vi "Main.vi"(0 "Operations Combo Box":string(combo)="Add", 1 "Load":bool, 5 "Add":bool, 7 "Delete":bool, 9 "Save":bool, 11 "error in":errorcluster, 12 "Tree":string(tree)) -> (15 "error out":errorcluster)   [LabVIEW 2023]
doc: "This is a simple calculator which can perform basic arithmetic operations like add, subtract, multiply and divide."
uses:
  Typedef/ClassClusters.ctl
  Arithmetic/Arithmetic.lvclass
  Typedef/InstancesArray.ctl
  Typedef/DVRcluster.ctl
  Typedef/DVRInstances.ctl
  Typedef/OperationsCluster.ctl
  Typedef/QueueOperations.ctl
  <vilib>/Utility/xml.llb/Write to XML File(string).vi
  <vilib>/Utility/xml.llb/Read From XML File(array).vi
panel:
  # "CALCULATOR"
  # "INSTRUCTIONS\n\n1. Run the VI.\n2. Choose the operations to perform from the Operations Combo Box.\n3. Press ADD to display once instance of the operations in the Tree.\n4. Press any instances in the tree to load that particular operations in \n    the subpanel.\n5. In the Sub-panel enter the inputs and press CALCULATE to get the \n     output.\n6. Press SAVE to save the operations data in the XML file.\n7. Press LOAD to retrive the save data from the XML, and press the saved\n    instance in the tree to display in the subpanel.\n8. Select any instance and press DELETE to reove from the tree.\n9. Close the Front panel to abort the VI."
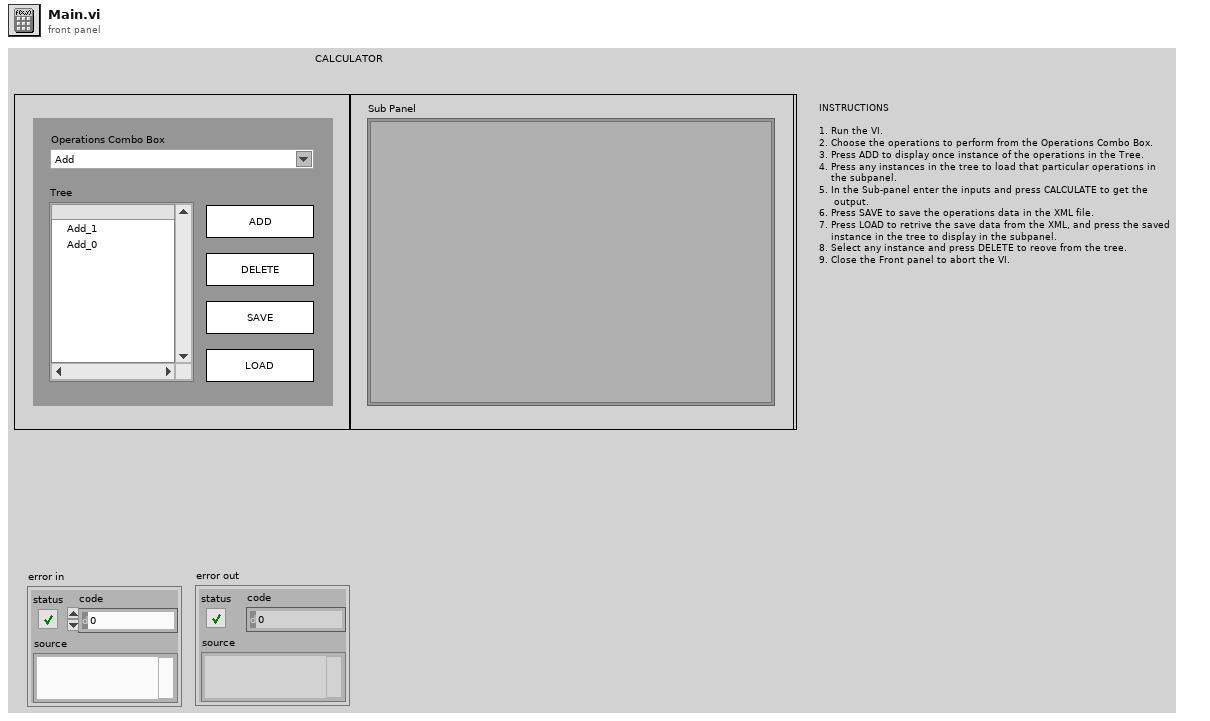
[diagram p1: front panel]
types:
  T1 = typedef "QueueOperations.ctl" = enum16{"Create", "Enqueue", "Enqueue N elements", "Dequeue", "Flush", "Release"}
  T2 = typedef "ClassClusters.ctl" = cluster{"Check":bool, "Combo Box":string, "Add":bool, "Delete":bool, "Path":path, "Tag":string, "Operation data":refnum<class "Arithmetic.lvclass">, "Instances Array":T3[], "XML path":path, "DVR":T4, "Operations Data":T6}
  T3 = typedef "InstancesArray.ctl" = cluster{"Tag":string, "Operation data":refnum<class "Arithmetic.lvclass">}
  T4 = typedef "DVRcluster.ctl" = cluster{"data value reference out":refnum<data-value>, "Operation Data DVR":refnum<data-value>, "Instances Array DVR":T5[]}
  T5 = typedef "DVRInstances.ctl" = cluster{"Operation Data DVR":refnum<data-value>, "Tag":string}
  T6 = typedef "OperationsCluster.ctl" = cluster{"A":dbl, "B":dbl, "C":dbl}
  T7 = typedef "LVPoint32TypeDef.ctl" = cluster{"Horizontal":i32, "Vertical":i32}
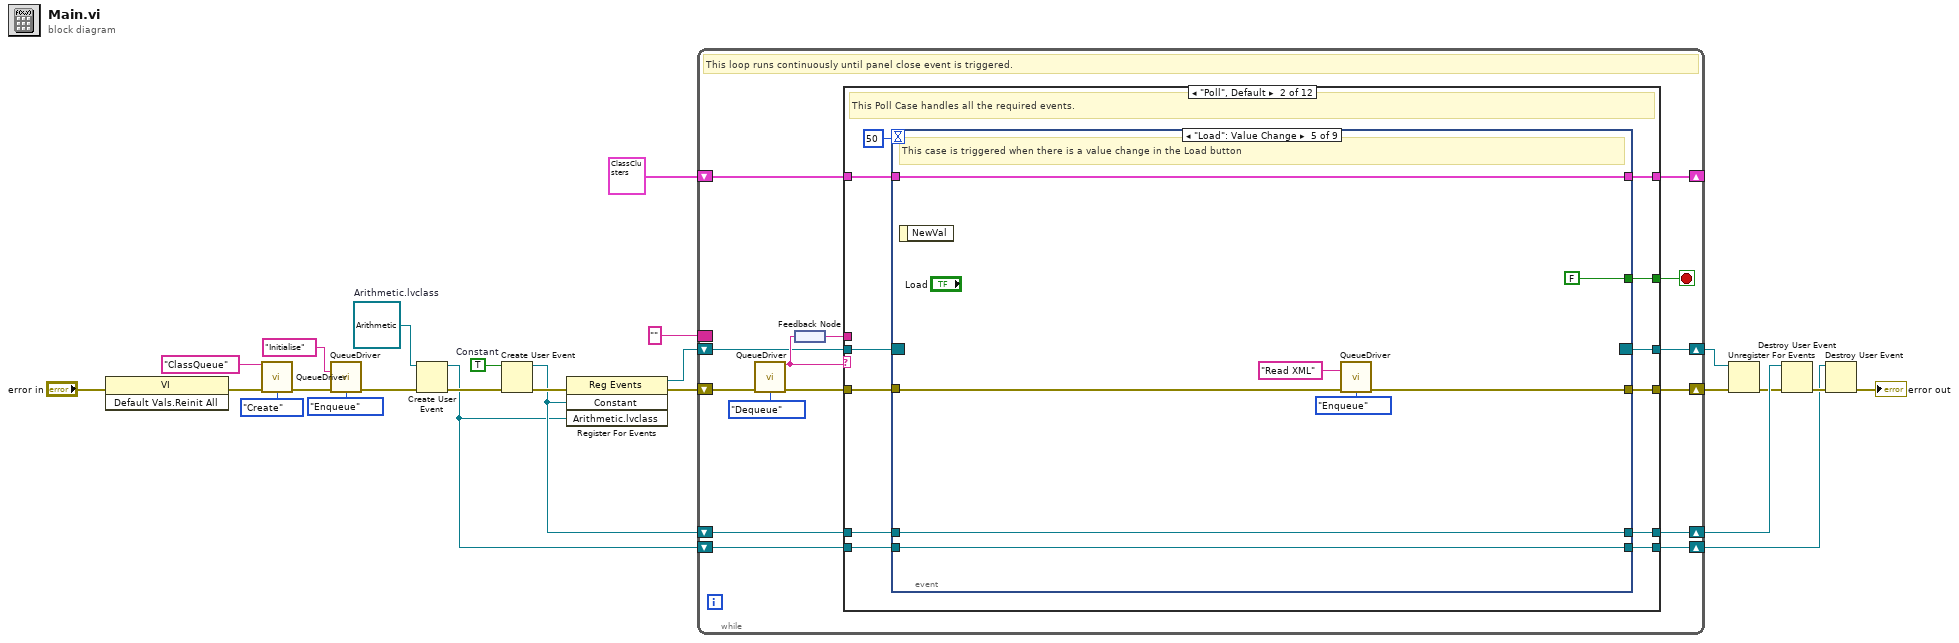
[diagram p0: block diagram]
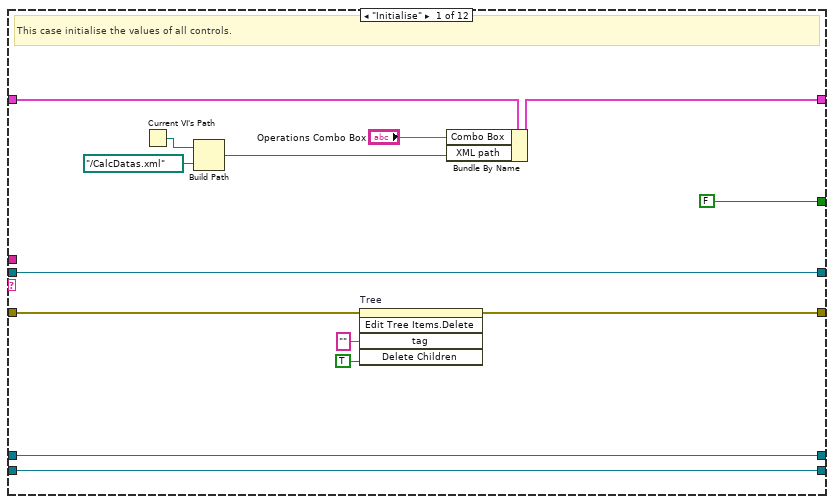
[diagram p2: hidden frame]
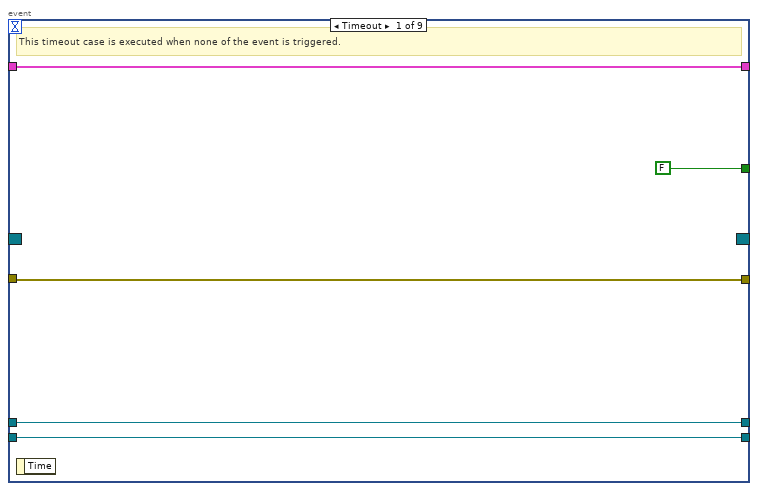
[diagram p3: hidden frame]
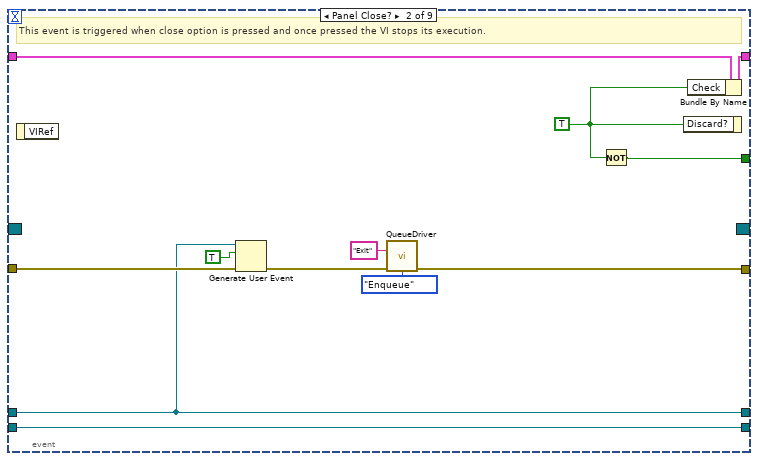
[diagram p4: hidden frame]
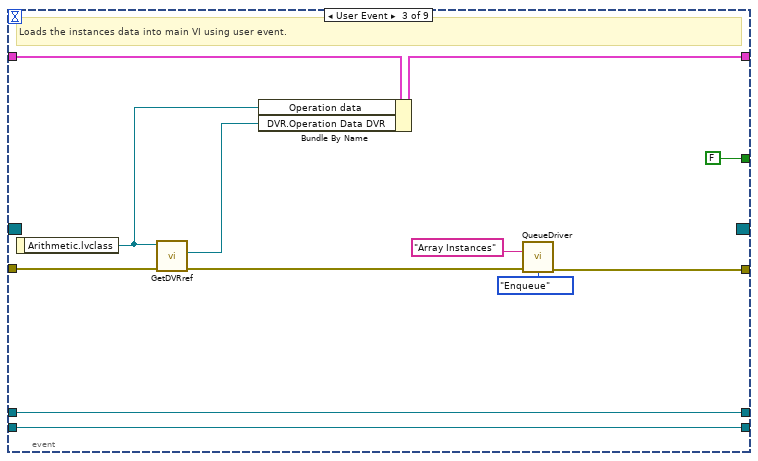
[diagram p5: hidden frame]
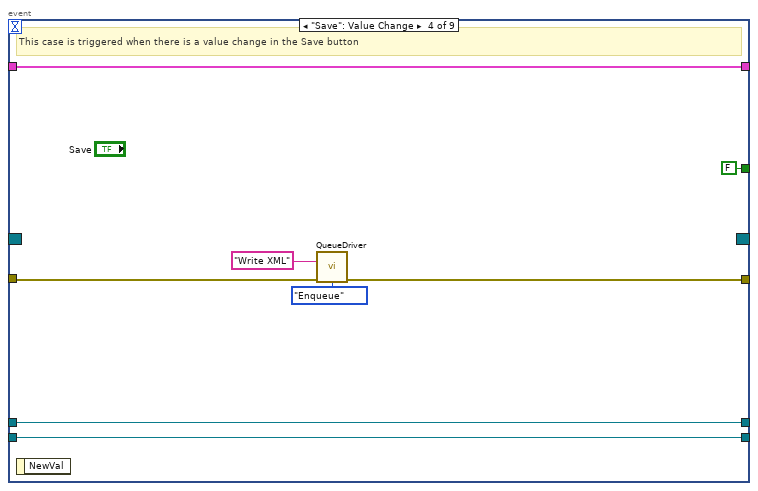
[diagram p6: hidden frame]
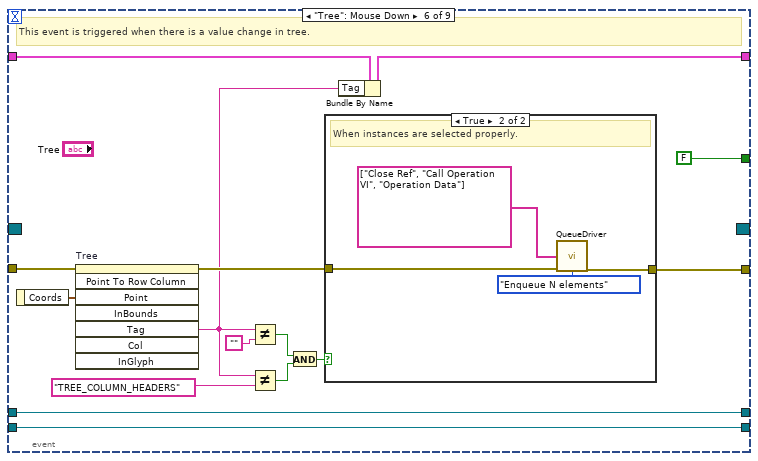
[diagram p7: hidden frame]
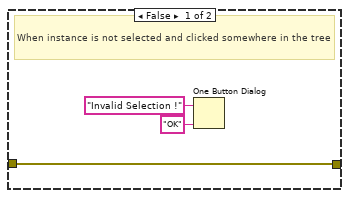
[diagram p8: hidden frame]
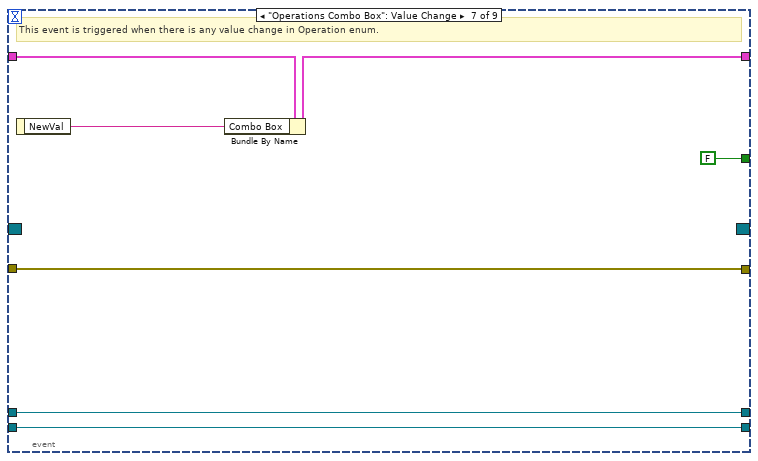
[diagram p9: hidden frame]
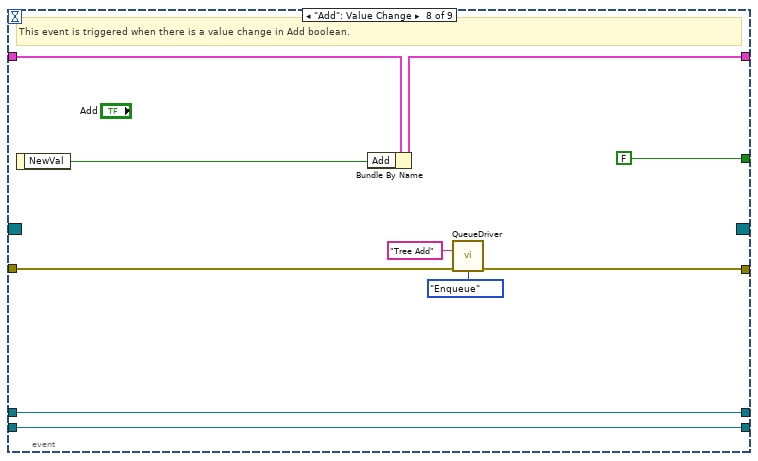
[diagram p10: hidden frame]
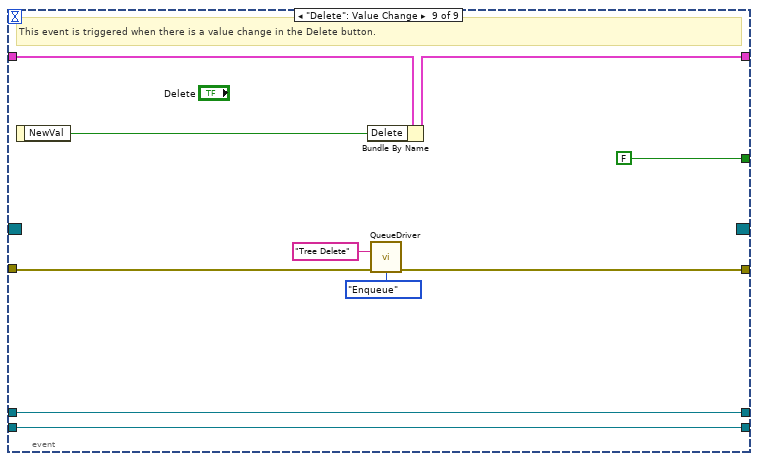
[diagram p11: hidden frame]
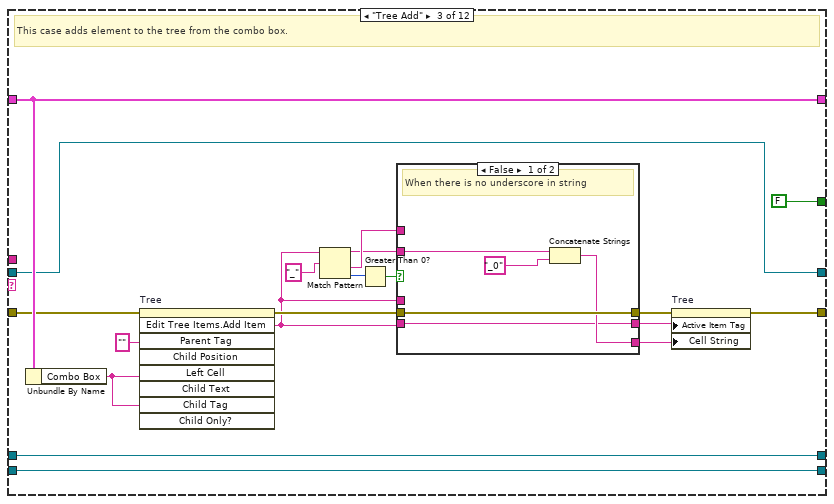
[diagram p12: hidden frame]
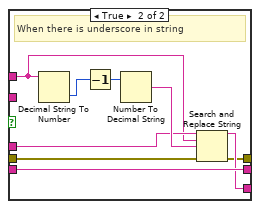
[diagram p13: hidden frame]
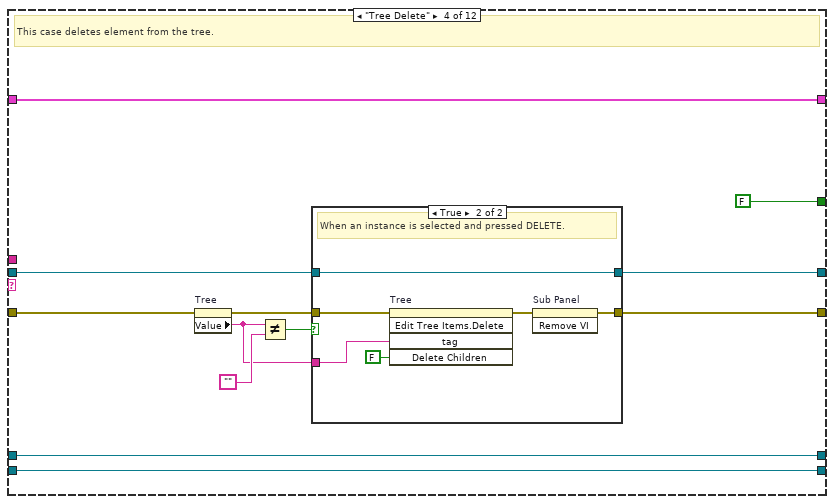
[diagram p14: hidden frame]
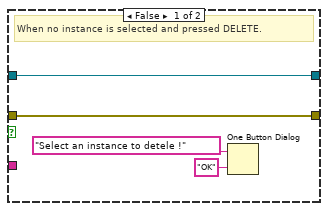
[diagram p15: hidden frame]
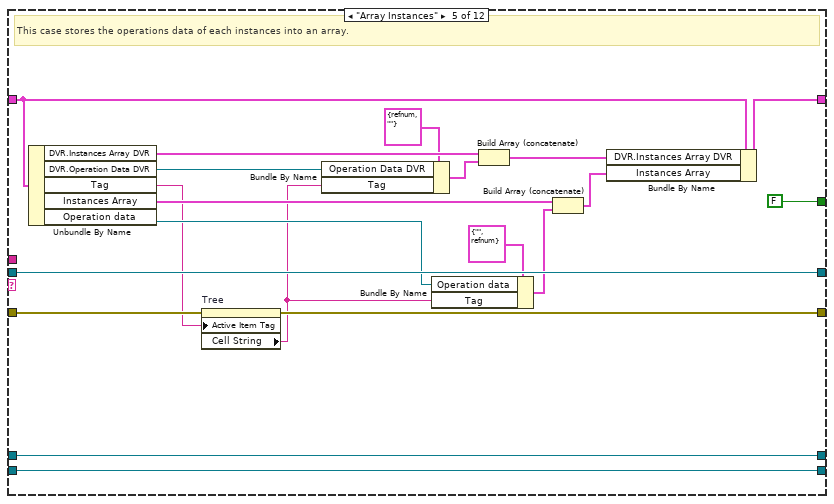
[diagram p16: hidden frame]
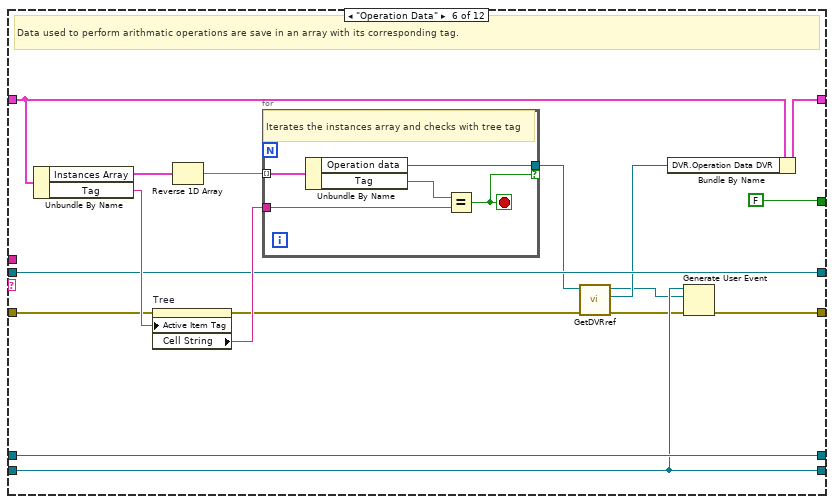
[diagram p17: hidden frame]
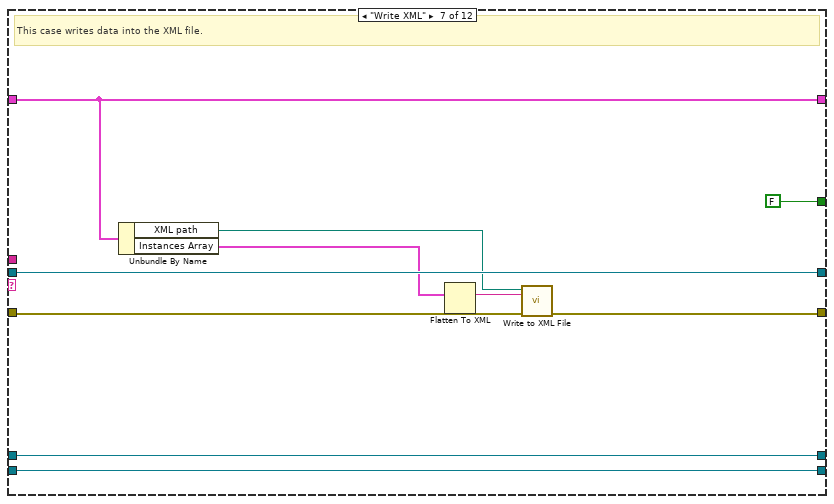
[diagram p18: hidden frame]
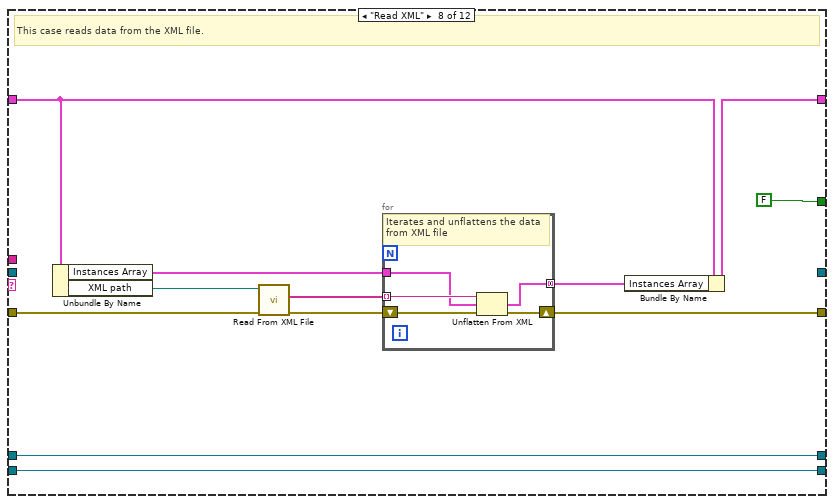
[diagram p19: hidden frame]
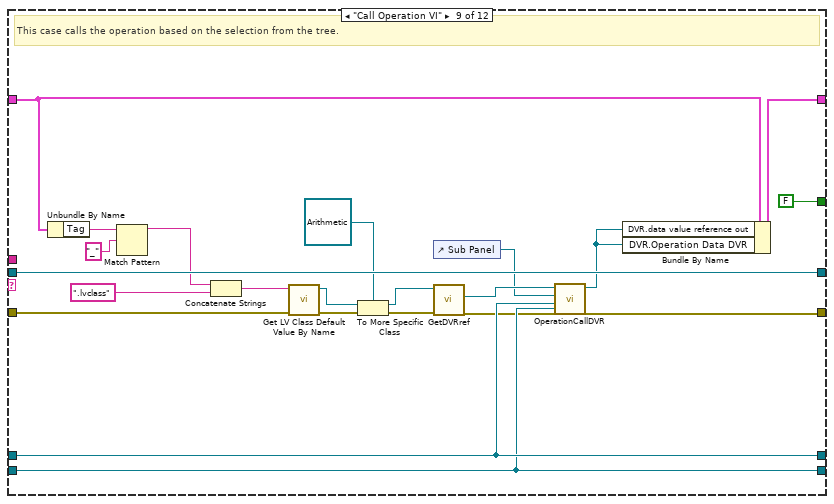
[diagram p20: hidden frame]
diagram:
  w5 = refnum<class "Arithmetic.lvclass"> refnum  # Arithmetic.lvclass
  w12 = TRUE  # Constant
  n1 = invoke class="VI" method="Default Vals.Reinit All"(error in="error in") -> (error out=w17:errorcluster)  [unwired: 2 in, 2 out]
  n2 = call "QueueDriver.vi"("Queue Name"="ClassQueue", "error in"=w17, "Queue Operations"=QueueOperations."Create") -> ("error out"=w24:errorcluster)  [unwired: 11 in, 1 out]
  n3 = call "QueueDriver.vi"("Enqueue State"="Initialise", "error in"=w24, "Queue Operations"=QueueOperations."Enqueue") -> ("error out"=w16:errorcluster)  [unwired: 11 in, 1 out]
  n4 = Create User Event(user event datatype=w5, error in=w16) -> (user event=w1:refnum<user-event>, error out=w15:errorcluster)
  n5 = Create User Event(user event datatype=w12, error in=w15) -> (user event=w10:refnum<user-event>, error out=w14:errorcluster)
  n6 = register-events(error in=w14, w10, w1) -> (reference out=w11:refnum<event-registration>, error out=w13:errorcluster)  [unwired: 1 in]
  n7 = while {
    shift-right: [w39] -> _
    shift-left: T2 {"Check"=FALSE, "Combo Box"="", "Add"=FALSE, "Delete"=FALSE, "Path"=path "", "Tag"="", "Operation data"=refnum, "Instances Array"=[], "XML path"=path "", "DVR"={"data value reference out"=refnum, "Operation Data DVR"=refnum, "Instances Array DVR"=[]}, "Operations Data"={"A"=0.0, "B"=0.0, "C"=0.0}} -> [w40]
    shift-right: [w35] -> w4
    shift-left: w13 -> [w38]
    border: "" ("Dequeue State") -> [_]
    shift-right: [w26] -> w2
    shift-left: w11 -> [w29]
    shift-right: [w28] -> w8
    shift-left: w10 -> [w31]
    shift-right: [w27] -> w6
    shift-left: w1 -> [w30]
    stop <- w32 stop-if-true
    # "This loop runs continuously until panel close event is triggered."
    n8 = call "QueueDriver.vi"("error in"=w38, "Queue Operations"=QueueOperations."Dequeue") -> ("Dequeue State"=w34:string, "error out"=w37:errorcluster)  [unwired: 12 in]
    n9 = feedback #1() -> (w33:string)
    n10 = feedback-in #1(w34) -> ()
    n11 = case shown="\"Poll\", Default" w34 {
      tunnel: w40 -> [w54 w66 w178 w204 w234 w246 w266 w277 w302 w309 w329 w339]
      tunnel: [w53 w65 w178 w204 w231 w244 w266 w273 w286 w309 w329 w339] -> w39
      tunnel: w37 -> [w50 w62 w177 w203 w232 w248 w260 w278 w303 w308 w319 w340]
      tunnel: [w43 w64 w172 w194 w227 w245 w259 w272 w287 w306 w320 w340] -> w35
      tunnel: w33 -> [_ _ _ _ _ _ _ _ _ _ w318 _]
      tunnel: [FALSE ("Check") w61 FALSE ("Check") FALSE ("Check") FALSE ("Check") FALSE ("Check") FALSE ("Check") FALSE ("Check") FALSE ("Check") FALSE ("Check") FALSE ("Check") w338] -> w32
      tunnel: w31 -> [w45 w60 w163 w200 w226 w243 w265 w271 w289 w313 w314 w337]
      tunnel: w30 -> [w46 w57 w164 w201 w225 w242 w264 w270 w288 w312 w315 w336]
      tunnel: w29 -> [w44 w59 w161 w196 w224 w241 w263 _ w304 w311 _ w335]
      tunnel: [w45 w58 w163 w200 w226 w243 w265 w271 w289 w313 w314 w337] -> w28
      tunnel: [w46 w56 w164 w201 w225 w242 w264 w270 w288 w312 w315 w336] -> w27
      tunnel: [w44 w55 w161 w195 w224 w241 w263 _ w304 w311 _ w335] -> w26
      frame "Initialise" {
        # "This case initialise the values of all controls."
        n12 = Current VI's Path() -> (path=w49:path)
        n13 = Build Path(base path=w49, name or relative path=path "../CalcDatas.xml") -> (appended path=w47:path)
        n14 = invoke on="Tree" class="Tree (strict)" method="Edit Tree Items.Delete"(error in=w50, "tag"="" ("Tag"), "Delete Children"=TRUE ("Delete Children?")) -> (error out=w43:errorcluster)  [unwired: 2 in, 4 out]
        n15 = Bundle By Name(cluster=w54, "Combo Box"="Operations Combo Box", "XML path"=w47) -> (w53:T2)
      }
      frame "Poll", Default {
        # "This Poll Case handles all the required events."
        n16 = event shown="[4] \"Load\": Value Change" {
          selector: w59 -> [_ _ _ _ _ _ _ _ _]
          dyn-events: [_ _ _ _ _ _ _ _ _] -> w55
          timeout: 50 -> [_ _ _ _ _ _ _ _ _]
          tunnel: w66 -> [w71 w83 w95 w103 w111 w126 w140 w150 w160]
          tunnel: [w71 w79 w93 w103 w111 w120 w139 w148 w158] -> w65
          tunnel: w62 -> [w70 w78 w86 w99 w107 w123 w136 w144 w154]
          tunnel: [w70 w81 w90 w98 w106 w125 w136 w143 w153] -> w64
          tunnel: [FALSE ("Check") w72 FALSE ("Check") FALSE ("Check") FALSE ("Check") FALSE ("Check") FALSE ("Check") FALSE ("Check") FALSE ("Check")] -> w61
          tunnel: w60 -> [w68 w75 w89 w97 w105 w118 w135 w142 w152]
          tunnel: [w68 w75 w89 w97 w105 w118 w135 w142 w152] -> w58
          tunnel: w57 -> [w67 w74 w88 w96 w104 w119 w134 w141 w151]
          tunnel: [w67 w74 w88 w96 w104 w119 w134 w141 w151] -> w56
          event Timeout {
            # "This timeout case is executed when none of the event is triggered."
            n17 = event-data() -> ()  [unwired: 1 in, 1 out]
          }
          event Panel Close? {
            w73 = TRUE ("Discard?")
            # "This event is triggered when close option is pressed and once pressed the VI stops its execution."
            n18 = event-data() -> ()  [unwired: 1 in, 1 out]
            n19 = Generate User Event(user event=w75, event data cluster=TRUE ("event data"), error in=w78) -> (error out=w77:errorcluster)  [unwired: 1 in, 1 out]
            n20 = call "QueueDriver.vi"("Enqueue State"="Exit", "error in"=w77, "Queue Operations"=QueueOperations."Enqueue") -> ("error out"=w81:errorcluster)  [unwired: 11 in, 1 out]
            n21 = Not(x=w73) -> (.not. x?=w72:bool)
            n22 = event-data("Discard?"=w73) -> ()  [unwired: 1 in, 1 out]
            n23 = Bundle By Name(cluster=w83, "Check"=w73) -> (w79:T2)
          }
          event User Event {
            # "Loads the instances data into main VI using user event."
            n24 = event-data() -> ("Arithmetic.lvclass"=w87:refnum<class "Arithmetic.lvclass">)  [unwired: 1 in]
            n25 = call-dynamic "GetDVRref.vi"("error in (no error)"=w86, "Arithmetic in"=w87) -> ("error out"=w85:errorcluster, "data value reference"=w84:refnum<data-value>)  [unwired: 6 in, 2 out]
            n26 = Bundle By Name(cluster=w95, "Operation data"=w87, "DVR.Operation Data DVR"=w84) -> (w93:T2)
            n27 = call "QueueDriver.vi"("Enqueue State"="Array Instances", "error in"=w85, "Queue Operations"=QueueOperations."Enqueue") -> ("error out"=w90:errorcluster)  [unwired: 11 in, 1 out]
          }
          event "Save": Value Change {
            # "This case is triggered when there is a value change in the Save button"
            n28 = event-data() -> ()  [unwired: 1 in, 1 out]
            n29 = call "QueueDriver.vi"("Enqueue State"="Write XML", "error in"=w99, "Queue Operations"=QueueOperations."Enqueue") -> ("error out"=w98:errorcluster)  [unwired: 11 in, 1 out]
          }
          event "Load": Value Change {
            # "This case is triggered when there is a value change in the Load button"
            n30 = event-data() -> ()  [unwired: 1 in, 1 out]
            n31 = call "QueueDriver.vi"("Enqueue State"="Read XML", "error in"=w107, "Queue Operations"=QueueOperations."Enqueue") -> ("error out"=w106:errorcluster)  [unwired: 11 in, 1 out]
          }
          event "Tree": Mouse Down {
            # "This event is triggered when there is a value change in tree."
            n32 = event-data() -> ("Coords"=w121:T7)  [unwired: 1 in]
            n33 = invoke on="Tree" class="Tree (strict)" method="Point To Row Column"(error in=w123, "Point"=w121) -> (error out=w122:errorcluster, "Tag"=w114:string)  [unwired: 6 in, 6 out]
            n34 = Not Equal?(x=w114, y="") -> (x != y?=w117:bool)
            n35 = Not Equal?(x=w114, y="TREE_COLUMN_HEADERS") -> (x != y?=w116:bool)
            n36 = And(x=w117, y=w116) -> (x .and. y?=w112:bool)
            n37 = case shown="True" w112 {
              tunnel: [w129 w132] -> w125
              tunnel: w122 -> [w129 w131]
              frame False {
                # "When instance is not selected and clicked somewhere in the tree"
                n38 = One Button Dialog(message="Invalid Selection !", button name ("OK")="OK") -> ()  [unwired: 1 out]
              }
              frame True {
                # "When instances are selected properly."
                n39 = call "QueueDriver.vi"("Array State"=string[] ["Close Ref", "Call Operation VI", "Operation Data"], "error in"=w131, "Queue Operations"=QueueOperations."Enqueue N elements") -> ("error out"=w132:errorcluster)  [unwired: 11 in, 1 out]
              }
            }
            n40 = Bundle By Name(cluster=w126, "Tag"=w114) -> (w120:T2)
          }
          event "Operations Combo Box": Value Change {
            # "This event is triggered when there is any value change in Operation enum."
            n41 = event-data() -> ("NewVal"=w137:string)  [unwired: 1 in]
            n42 = Bundle By Name(cluster=w140, "Combo Box"=w137) -> (w139:T2)
          }
          event "Add": Value Change {
            # "This event is triggered when there is a value change in Add boolean."
            n43 = event-data() -> ("NewVal"=w147:bool)  [unwired: 1 in]
            n44 = Bundle By Name(cluster=w150, "Add"=w147) -> (w148:T2)
            n45 = call "QueueDriver.vi"("Enqueue State"="Tree Add", "error in"=w144, "Queue Operations"=QueueOperations."Enqueue") -> ("error out"=w143:errorcluster)  [unwired: 11 in, 1 out]
          }
          event "Delete": Value Change {
            # "This event is triggered when there is a value change in the Delete button."
            n46 = event-data() -> ("NewVal"=w157:bool)  [unwired: 1 in]
            n47 = Bundle By Name(cluster=w160, "Delete"=w157) -> (w158:T2)
            n48 = call "QueueDriver.vi"("Enqueue State"="Tree Delete", "error in"=w154, "Queue Operations"=QueueOperations."Enqueue") -> ("error out"=w153:errorcluster)  [unwired: 11 in, 1 out]
          }
        }
      }
      frame "Tree Add" {
        # "This case adds element to the tree from the combo box."
        n49 = Unbundle By Name(w178) -> ("Combo Box"=w176:string)
        n50 = invoke on="Tree" class="Tree (strict)" method="Edit Tree Items.Add Item"(error in=w177, "Parent Tag"="", "Left Cell"=w176, "Child Tag"=w176) -> (error out=w174:errorcluster, "Edit Tree Items:Add Item"=w168:string)  [unwired: 5 in, 7 out]
        n51 = Match Pattern(string=w168, regular expression="_") -> (before substring=w166:string, after substring=w167:string, offset past match=w171:i32)  [unwired: 1 in, 1 out]
        n52 = Greater Than 0?(x=w171) -> (x > 0?=w170:bool)
        n53 = case shown="False" w170 {
          tunnel: w174 -> [w184 w186]
          tunnel: [w184 w185] -> w173
          tunnel: w168 -> [w181 w193]
          tunnel: [w181 w193] -> w162
          tunnel: [w182 w189] -> w169
          tunnel: w168 -> [_ w190]
          tunnel: w166 -> [w180 _]
          tunnel: w167 -> [_ w188]
          frame False {
            # "When there is no underscore in string"
            n54 = Concatenate Strings(w180, "_0" ("string")) -> (w182:string)
          }
          frame True {
            # "When there is underscore in string"
            n55 = Decimal String To Number(string=w188) -> (number=w187:i32)  [unwired: 2 in, 1 out]
            n56 = Decrement(x=w187) -> (x-1=w192:i32)
            n57 = Number To Decimal String(number=w192) -> (decimal integer string=w191:string)  [unwired: 1 in]
            n58 = Search and Replace String(input string=w190, search string=w188, replace string=w191, error in=w186) -> (result string=w189:string, error out=w185:errorcluster)  [unwired: 4 in, 2 out]
          }
        }
        n59 = property on="Tree" class="Tree (strict)"(error in=w173, "Active Item Tag"=w162, "Cell String"=w169) -> (error out=w172:errorcluster)  [unwired: 1 in, 1 out]
      }
      frame "Tree Delete" {
        # "This case deletes element from the tree."
        n60 = property on="Tree" class="Tree (strict)"(error in=w203) -> (error out=w202:errorcluster, "Value"=w197:string)  [unwired: 1 in, 1 out]
        n61 = Not Equal?(x=w197, y="") -> (x != y?=w198:bool)
        n62 = case shown="True" w198 {
          tunnel: w202 -> [w208 w215]
          tunnel: [w208 w210] -> w194
          tunnel: w197 -> [_ w213]
          tunnel: w196 -> [w209 w212]
          tunnel: [w209 w212] -> w195
          frame False {
            # "When no instance is selected and pressed DELETE."
            n63 = One Button Dialog(message="Select an instance to detele !", button name ("OK")="OK") -> ()  [unwired: 1 out]
          }
          frame True {
            # "When an instance is selected and pressed DELETE."
            n64 = invoke on="Tree" class="Tree (strict)" method="Edit Tree Items.Delete"(error in=w215, "tag"=w213, "Delete Children"=FALSE ("Delete Children?")) -> (error out=w211:errorcluster)  [unwired: 2 in, 4 out]
            n65 = invoke on="Sub Panel" class="SubPnl" method="Remove VI"(error in=w211) -> (error out=w210:errorcluster)  [unwired: 2 in, 2 out]
          }
        }
      }
      frame "Array Instances" {
        # "This case stores the operations data of each instances into an array."
        n66 = Unbundle By Name(w234) -> ("DVR.Instances Array DVR"=w230:T5[], "DVR.Operation Data DVR"=w233:refnum<data-value>, "Tag"=w217:string, "Instances Array"=w219:T3[], "Operation data"=w221:refnum<class "Arithmetic.lvclass">)
        n67 = property on="Tree" class="Tree (strict)"(error in=w232, "Active Item Tag"=w217) -> (error out=w227:errorcluster, "Cell String"=w216:string)  [unwired: 1 in, 1 out]
        n68 = Bundle By Name(cluster=T5 {"Operation Data DVR"=refnum, "Tag"=""} ("DVR Instances"), "Operation Data DVR"=w233, "Tag"=w216) -> (w229:T5)
        n69 = Bundle By Name(cluster=T3 {"Tag"="", "Operation data"=refnum} ("Cluster"), "Operation data"=w221, "Tag"=w216) -> (w220:T3)
        n70 = Build Array (concatenate)(w230, w229) -> (w228:T5[])
        n71 = Build Array (concatenate)(w219, w220) -> (w218:T3[])
        n72 = Bundle By Name(cluster=w234, "DVR.Instances Array DVR"=w228, "Instances Array"=w218) -> (w231:T2)
      }
      frame "Operation Data" {
        # "Data used to perform arithmatic operations are save in an array with its corresponding tag."
        n73 = Unbundle By Name(w246) -> ("Instances Array"=w251:T3[], "Tag"=w249:string)
        n74 = property on="Tree" class="Tree (strict)"(error in=w248, "Active Item Tag"=w249) -> (error out=w240:errorcluster, "Cell String"=w247:string)  [unwired: 1 in, 1 out]
        n75 = Reverse 1D Array(array=w251) -> (reversed array=w250:T3[])
        n76 = for {
          tunnel: w250 -> [w257] mode=indexing
          tunnel: w247 -> [w256]
          tunnel: [w254] -> w238 if=w253
          stop <- w253 stop-if-true
          # "Iterates the instances array and checks with tree tag"
          n77 = Unbundle By Name(w257) -> ("Operation data"=w254:refnum<class "Arithmetic.lvclass">, "Tag"=w255:string)
          n78 = Equal?(x=w255, y=w256) -> (x = y?=w253:bool)
        }
        n79 = call-dynamic "GetDVRref.vi"("error in (no error)"=w240, "Arithmetic in"=w238) -> ("error out"=w239:errorcluster, "data value reference"=w237:refnum<data-value>, "Arithmetic out"=w236:refnum<class "Arithmetic.lvclass">)  [unwired: 6 in, 1 out]
        n80 = Bundle By Name(cluster=w246, "DVR.Operation Data DVR"=w237) -> (w244:T2)
        n81 = Generate User Event(user event=w242, event data cluster=w236, error in=w239) -> (error out=w245:errorcluster)  [unwired: 1 in, 1 out]
      }
      frame "Write XML" {
        # "This case writes data into the XML file."
        n82 = Unbundle By Name(w266) -> ("XML path"=w258:path, "Instances Array"=w261:T3[])
        n83 = Flatten To XML(6:w261) -> (2:w262:string)
        n84 = call-poly <vilib>:"Write to XML File.vi"("error in (no error)"=w260, "XML Input"=w262, "XML File Path"=w258) -> ("error out"=w259:errorcluster)  [unwired: 6 in, 2 out]
      }
      frame "Read XML" {
        # "This case reads data from the XML file."
        n85 = Unbundle By Name(w277) -> ("Instances Array"=w269:T3[], "XML path"=w276:path)
        n86 = call-poly <vilib>:"Read From XML File.vi"("error in (no error)"=w278, "XML File Path"=w276) -> ("error out"=w274:errorcluster, "XML Elements"=w275:string[])  [unwired: 7 in, 1 out]
        n87 = for {
          tunnel: w275 -> [w284] mode=indexing
          shift-right: [w282] -> w272
          shift-left: w274 -> [w283]
          tunnel: w269 -> [w281]
          tunnel: [w280] -> w268 mode=concatenating
          # "Iterates and unflattens the data from XML file"
          n88 = Unflatten From XML(xml string=w284, type=w281, error in (no error)=w283) -> (value=w280:T3[], error out=w282:errorcluster)
        }
        n89 = Bundle By Name(cluster=w277, "Instances Array"=w268) -> (w273:T2)
      }
      frame "Call Operation VI" {
        # "This case calls the operation based on the selection from the tree."
        n90 = Unbundle By Name(w302) -> ("Tag"=w297:string)
        n91 = Match Pattern(string=w297, regular expression="_") -> (before substring=w296:string)  [unwired: 1 in, 3 out]
        n92 = Concatenate Strings(w296, ".lvclass" ("string")) -> (w301:string)
        n93 = call <vilib>:"Get LV Class Default Value By Name.vi"("error in (no error)"=w303, "class name"=w301) -> ("error out"=w299:errorcluster, "object"=w298:refnum<class>)  [unwired: 8 in]
        n94 = To More Specific Class(target class=refnum<class "Arithmetic.lvclass"> refnum ("Parent Class"), reference=w298, error in=w299) -> (specific class reference=w293:refnum<class "Arithmetic.lvclass">, error out=w292:errorcluster)
        n95 = control-ref of="Sub Panel"() -> (w290:refnum<vi>)
        n96 = call-dynamic "GetDVRref.vi"("error in (no error)"=w292, "Arithmetic in"=w293) -> ("error out"=w287:errorcluster, "data value reference"=w291:refnum<data-value>)  [unwired: 6 in, 2 out]
        n97 = call "OperationCallDVR.vi"("event source"=w288, "user event out"=w289, "Sub Panel"=w290, "data value reference in"=w291) -> ("data value reference out"=w285:refnum<data-value>)  [unwired: 7 in]
        n98 = Bundle By Name(cluster=w302, "DVR.data value reference out"=w285, "DVR.Operation Data DVR"=w285) -> (w286:T2)
      }
      frame "Close Ref" {
        # "Closes the DVR reference."
        n99 = Unbundle By Name(w309) -> ("DVR.data value reference out"=w307:refnum<data-value>)
        n100 = call "CloseRefDVR.vi"("error in (no error)"=w308, "data value reference in"=w307) -> ("error out"=w306:errorcluster)  [unwired: 8 in, 1 out]
      }
      frame "Error" {
        # "This case handles the error."
        n101 = Unbundle By Name(w319) -> ("code"=w317:i32, "source"=w321:string)
        n102 = call <vilib>:"Clear Errors.vi"("error in (no error)"=w319, "specific error code to clear (0: all)"=w317) -> ("error out"=w325:errorcluster)  [unwired: 4 in, 1 out]
        n103 = Format Into String(format string="Error occurred in state \"%s\"!!\nError Code: %d\nError Source: %s\n\nDo you wish to continue?", error in=w325, w318, w317, w321) -> (resulting string=w326:string, error out=w328:errorcluster)  [unwired: 1 in]
        n104 = Two Button Dialog(message=w326, 1:"Exit" ("F button name (\"Cancel\")"), 2:"Continue" ("T button name (\"OK\")")) -> (T button?=w327:bool)
        n105 = case shown="False" w327 {
          tunnel: w328 -> [w331 w334]
          tunnel: [w330 w334] -> w320
          frame False {
            # "Exit"
            n106 = call "QueueDriver.vi"("Enqueue State"="Exit", "error in"=w331, "Queue Operations"=QueueOperations."Enqueue") -> ("error out"=w330:errorcluster)  [unwired: 11 in, 1 out]
          }
          frame True {
            # "Continue"
          }
        }
      }
      frame "Exit" {
        # "This case is handled when the panel close event is triggered."
        n107 = Unbundle By Name(w339) -> ("Check"=w338:bool)
      }
    }
  }
  n108 = Unregister For Events(event registration refnum=w2, error in=w4) -> (error out=w3:errorcluster)
  n109 = Destroy User Event(user event=w8, error in=w3) -> (error out=w9:errorcluster)
  n110 = Destroy User Event(user event=w6, error in=w9) -> (error out=→"error out":errorcluster)
